vi "主界面.vi"() -> ()   [LabVIEW 2010]
panel:
  in  "余额":bool
  out "字符串":string
  in  "退出":bool
  in  "出账":bool
  in  "进账":bool
  # "个人小金库系统"
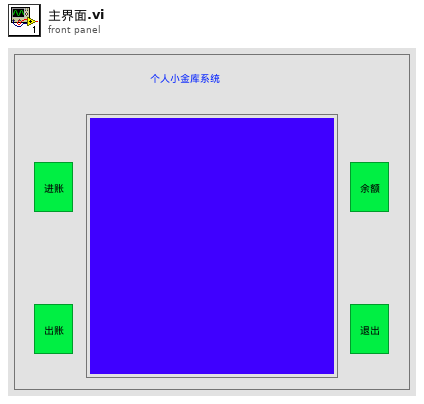
[diagram p1: front panel]
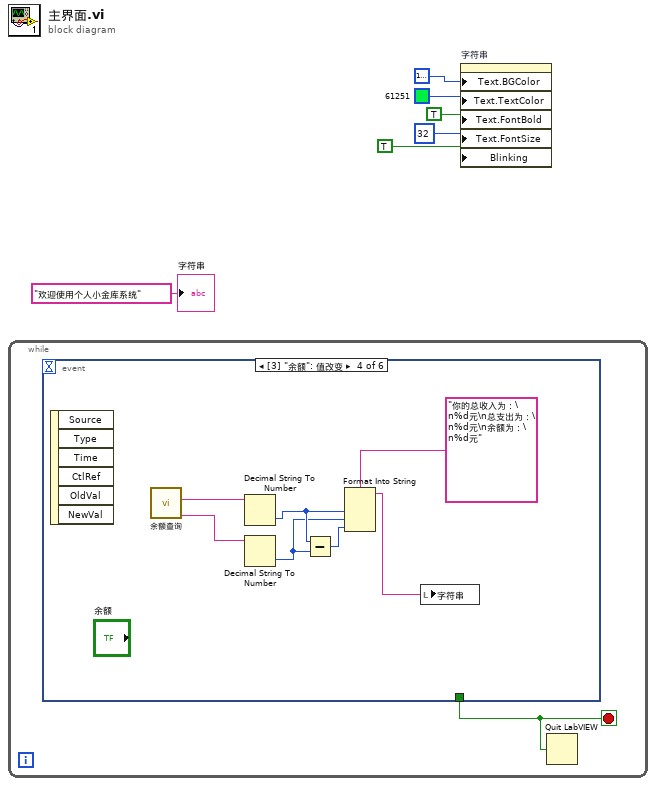
[diagram p0: block diagram]
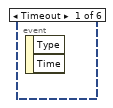
[diagram p2: hidden frame]
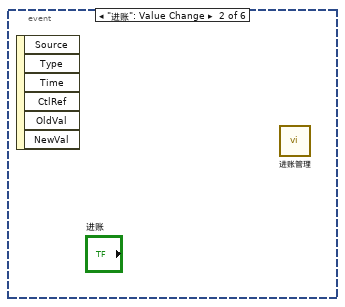
[diagram p3: hidden frame]
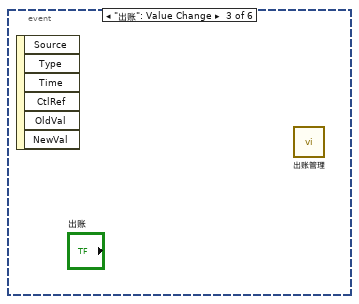
[diagram p4: hidden frame]
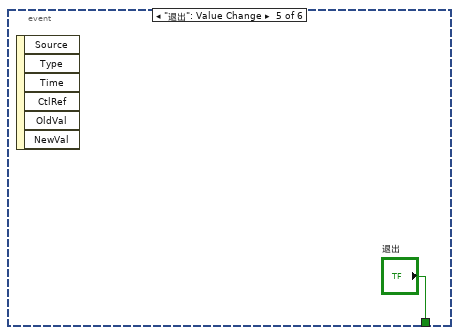
[diagram p5: hidden frame]
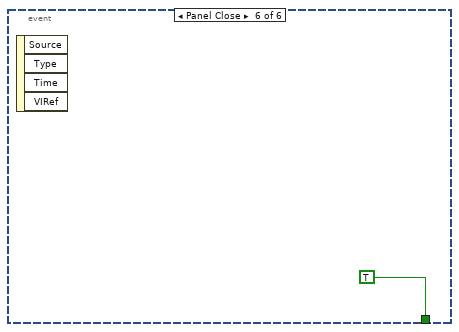
[diagram p6: hidden frame]
diagram:
  n1 = while {
    stop <- w7 stop-if-true
    n2 = event shown="[3] \"余额\": 值改变" {
      selector: _ -> [_ _ _ _ _ _]
      dyn-events: _ -> [_ _ _ _ _ _]
      timeout: _ -> [_ _ _ _ _ _]
      tunnel: [_ _ _ _ "退出" TRUE] -> w7
      event Timeout {
        n3 = event-data() -> ()  [unwired: 1 in, 2 out]
      }
      event "进账": Value Change {
        n4 = event-data() -> ()  [unwired: 1 in, 6 out]
        n5 = call "进账管理.vi"() -> ()  [unwired: 1 in]
      }
      event "出账": Value Change {
        n6 = event-data() -> ()  [unwired: 1 in, 6 out]
        n7 = call "出账管理.vi"() -> ()  [unwired: 1 in]
      }
      event "余额": Value Change {
        n8 = event-data() -> ()  [unwired: 1 in, 6 out]
        n9 = call "余额查询.vi"() -> ("出账总额"=w11:string, "进账总额"=w12:string)  [unwired: 10 in]
        n10 = Decimal String To Number(string=w12) -> (number=w10:i32)  [unwired: 2 in, 1 out]
        n11 = Decimal String To Number(string=w11) -> (number=w9:i32)  [unwired: 2 in, 1 out]
        n12 = Subtract(x=w10, y=w9) -> (x-y=w8:i32)
        n13 = Format Into String(format string="你的总收入为：\n%d元\n总支出为：\n%d元\n余额为：\n%d元", w10, w9, w8) -> (resulting string=w13:string)  [unwired: 2 in, 1 out]
        n14 = local write "字符串"(w13) -> ()
      }
      event "退出": Value Change {
        n15 = event-data() -> ()  [unwired: 1 in, 6 out]
      }
      event Panel Close {
        n16 = event-data() -> ()  [unwired: 1 in, 4 out]
      }
    }
    n17 = Quit LabVIEW(quit? (T)=w7) -> ()
  }
  n18 = property on="字符串" class="Str"("Text.BGColor"=u32 16777228, "Text.TextColor"=u32 61251, "Text.FontBold"=TRUE ("文本.字体:粗体"), "Text.FontSize"=u32 32 ("文本.字体:字号"), "Blinking"=TRUE ("闪烁")) -> ()  [unwired: 2 in, 2 out]
  "字符串" <- "欢迎使用个人小金库系统"
